vi "EstimateTargetingInformation.vi"(0 "X (in) [t0]":dbl, 1 "Y (in) [t0]":dbl, 5 "Turret Heading (deg)":dbl, 7 "Robot Heading (deg)":dbl, 8 "Velocity Magnitude (ft/s)":dbl, 9 "Far Acceptable Heading Error (deg)":dbl=4.0, 10 "Velocity Heading (deg)":dbl, 11 "Close Acceptable Heading Error (deg)":dbl=4.0, 12 "Vision Horizontal Angle to Target (deg) [t-?]":dbl, 13 "Min Timed Aligned (ms)":u32=500, 15 "Angular Target Shift (deg)":dbl, 17 "Radial Target Shift (in)":dbl) -> (20 "Fused Distance to Target (in)":dbl, 21 "Fused Heading to Target (deg)":dbl, 23 "Pointed At Target":bool, 24 "Pointing Angle Error (deg)":dbl format="%_4g", 25 "Targeting Predictions":dbl[](array[numeric]))   [LabVIEW 2020]
doc: "This VI estimates the shooter's heading and range to the target based on the current and projected robot pose."
uses:
  robotconstants.vi
  drivercommands.vi
  driverdata.vi
  robotoutputs.vi
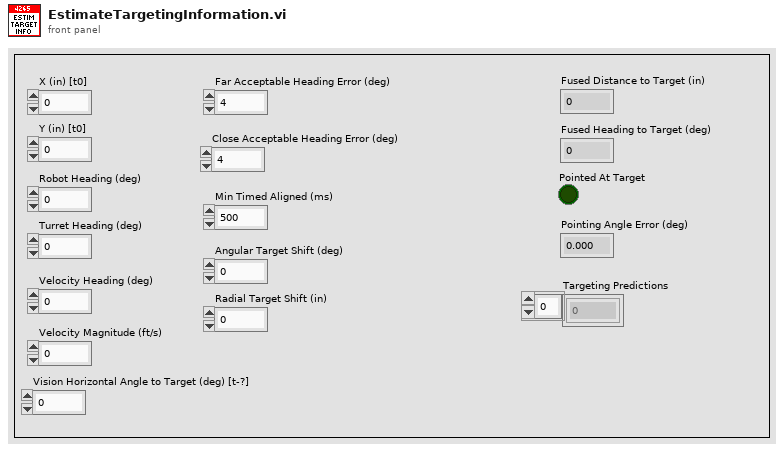
[diagram p1: front panel]
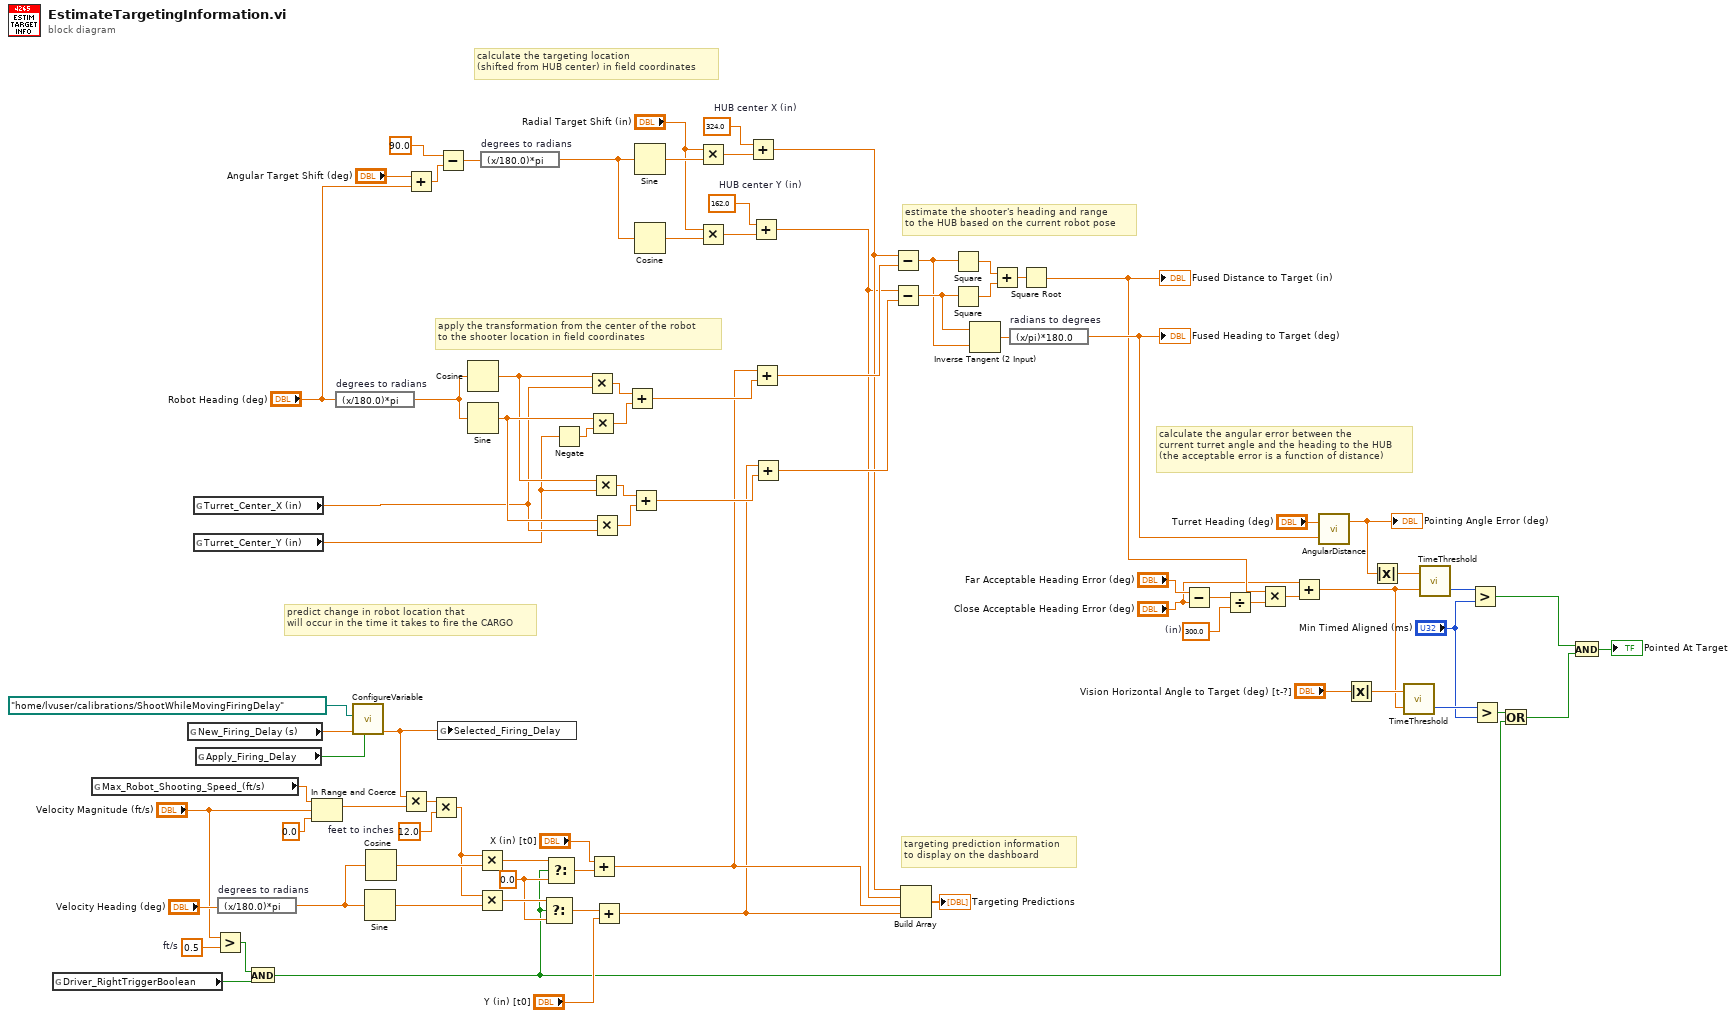
[diagram p0: block diagram]
diagram:
  w20 = 300.0  # (in)
  w35 = 0.5  # ft/s
  w37 = 0.0 ("f")
  w41 = 12.0  # feet to inches
  w49 = 162.0  # HUB center Y (in)
  w52 = 324.0  # HUB center X (in)
  # "predict change in robot location that\nwill occur in the time it takes to fire the CARGO"
  # "targeting prediction information\nto display on the dashboard"
  # "calculate the targeting location\n(shifted from HUB center) in field coordinates"
  # "apply the transformation from the center of the robot\nto the shooter location in field coordinates"
  # "calculate the angular error between the\ncurrent turret angle and the heading to the HUB\n(the acceptable error is a function of distance)"
  # "estimate the shooter's heading and range\nto the HUB based on the current robot pose"
  n1 = global read "drivercommands.vi" "Driver_RightTriggerBoolean"() -> (w24:bool)
  n2 = global read "robotconstants.vi" "Max_Robot_Shooting_Speed_(ft/s)"() -> (w27:dbl)
  n3 = global read "driverdata.vi" "New_Firing_Delay (s)"() -> (w13:dbl)
  n4 = global read "robotconstants.vi" "Turret_Center_X (in)"() -> (w71:dbl)
  n5 = global read "robotconstants.vi" "Turret_Center_Y (in)"() -> (w70:dbl)
  n6 = global read "driverdata.vi" "Apply_Firing_Delay"() -> (w12:bool)
  n7 = Greater?(x="Velocity Magnitude (ft/s)", y=w35) -> (0:w23:bool)
  n8 = expression code="(x/180.0)*pi" "degrees to radians"("Velocity Heading (deg)") -> (w45:dbl)
  n9 = And(x=w23, y=w24) -> (x .and. y?=w2:bool)
  n10 = In Range and Coerce(upper limit=w27, x="Velocity Magnitude (ft/s)", lower limit=0.0 ("x")) -> (coerced(x)=w25:dbl)  [unwired: 1 out]
  n11 = expression code="(x/180.0)*pi" "degrees to radians"("Robot Heading (deg)") -> (w72:dbl)
  n12 = call "ConfigureVariable.vi"("Apply New Setpoint"=w12, "New Setpoint Value"=w13, "Setpoint Save Location"=path "/home/lvuser/calibrations/ShootWhileMovingFiringDelay") -> ("Selected Setpoint Value"=w22:dbl)  [unwired: 8 in]
  n13 = Sine(x=w45) -> (sin(x)=w43:dbl)
  n14 = Cosine(x=w45) -> (cos(x)=w44:dbl)
  n15 = Multiply(x=w22, y=w25) -> (x*y=w42:dbl)
  n16 = Add(x="Angular Target Shift (deg)", y="Robot Heading (deg)") -> (x+y=w60:dbl)
  n17 = Multiply(x=w42, y=w41) -> (x*y=w40:dbl)
  n18 = Subtract(x=90.0, y=w60) -> (x-y=w57:dbl)
  n19 = global write "robotoutputs.vi" "Selected_Firing_Delay"(w22) -> ()
  n20 = Cosine(x=w72) -> (cos(x)=w78:dbl)
  n21 = Sine(x=w72) -> (sin(x)=w79:dbl)
  n22 = Multiply(x=w40, y=w44) -> (x*y=w39:dbl)
  n23 = Multiply(x=w40, y=w43) -> (x*y=w38:dbl)
  n24 = expression code="(x/180.0)*pi" "degrees to radians"(w57) -> (w55:dbl)
  n25 = Select(t=w38, s=w2, f=w37) -> (s? t:f=w34:dbl)
  n26 = Select(t=w39, s=w2, f=w37) -> (s? t:f=w32:dbl)
  n27 = Negate(x=w70) -> (-x=w73:dbl)
  n28 = Multiply(x=w78, y=w71) -> (x*y=w74:dbl)
  n29 = Multiply(x=w79, y=w73) -> (x*y=w75:dbl)
  n30 = Add(x="X (in) [t0]", y=w32) -> (x+y=w30:dbl)
  n31 = Multiply(x=w78, y=w70) -> (x*y=w76:dbl)
  n32 = Multiply(x=w79, y=w71) -> (x*y=w77:dbl)
  n33 = Add(x=w34, y="Y (in) [t0]") -> (x+y=w29:dbl)
  n34 = Add(x=w74, y=w75) -> (x+y=w69:dbl)
  n35 = Add(x=w76, y=w77) -> (x+y=w68:dbl)
  n36 = Sine(x=w55) -> (sin(x)=w56:dbl)
  n37 = Cosine(x=w55) -> (cos(x)=w54:dbl)
  n38 = Multiply(x="Radial Target Shift (in)", y=w56) -> (x*y=w51:dbl)
  n39 = Multiply(x="Radial Target Shift (in)", y=w54) -> (x*y=w50:dbl)
  n40 = Add(x=w52, y=w51) -> (x+y=w48:dbl)
  n41 = Add(x=w49, y=w50) -> (x+y=w47:dbl)
  n42 = Add(x=w30, y=w69) -> (x+y=w65:dbl)
  n43 = Add(x=w29, y=w68) -> (x+y=w64:dbl)
  n44 = Subtract(x=w48, y=w65) -> (x-y=w66:dbl)
  n45 = Subtract(x=w47, y=w64) -> (x-y=w67:dbl)
  n46 = Build Array(w48, w47, w30, w29) -> (→"Targeting Predictions":dbl[])
  n47 = Square(x=w66) -> (x^2=w85:dbl)
  n48 = Square(x=w67) -> (x^2=w84:dbl)
  n49 = Inverse Tangent (2 Input)(1:w66, 2:w67) -> (0:w82:dbl)
  n50 = Add(x=w85, y=w84) -> (x+y=w83:dbl)
  n51 = expression code="(x/pi)*180.0" "radians to degrees"(w82) -> (w28:dbl)
  "Fused Heading to Target (deg)" <- w28
  n52 = Square Root(x=w83) -> (sqrt(x)=w18:dbl)
  "Fused Distance to Target (in)" <- w18
  n53 = Subtract(x="Far Acceptable Heading Error (deg)", y="Close Acceptable Heading Error (deg)") -> (x-y=w21:dbl)
  n54 = Divide(x=w21, y=w20) -> (x/y=w19:dbl)
  n55 = Multiply(x=w18, y=w19) -> (x*y=w17:dbl)
  n56 = Add(x="Close Acceptable Heading Error (deg)", y=w17) -> (x+y=w1:dbl)
  n57 = call "AngularDistance.vi"("Goal Angle (deg) [0,360]"=w28, "Current Angle (deg) [-Inf,+Inf]"="Turret Heading (deg)") -> ("Signed Angular Distance (deg) [-180,+180]"=w63:dbl)  [unwired: 1 out]
  "Pointing Angle Error (deg)" <- w63
  n58 = Absolute Value(x="Vision Horizontal Angle to Target (deg) [t-?]") -> (abs(x)=w9:dbl)
  n59 = Absolute Value(x=w63) -> (abs(x)=w81:dbl)
  n60 = call "TimeThreshold.vi"("Threshold"=w1, "Current Value"=w9) -> ("Time Below Threshold (ms)"=w8:u32)  [unwired: 1 out]
  n61 = call "TimeThreshold.vi"("Threshold"=w1, "Current Value"=w81) -> ("Time Below Threshold (ms)"=w80:u32)  [unwired: 1 out]
  n62 = Greater?(x=w80, y="Min Timed Aligned (ms)") -> (0:w5:bool)
  n63 = Greater?(x=w8, y="Min Timed Aligned (ms)") -> (0:w4:bool)
  n64 = Or(x=w4, y=w2) -> (x .or. y?=w3:bool)
  n65 = And(x=w5, y=w3) -> (x .and. y?=→"Pointed At Target":bool)
